vi "Delete Tags.vi"(8 "error in (no error)":errorcluster, 10 "Tag":string[](array[string]), 11 "Tag Tree In":refnum<class "Tag Tree.lvclass">) -> (0 "error out":errorcluster, 3 "Tag Tree Out":refnum<class "Tag Tree.lvclass">)   [LabVIEW 2020, in "Tag Tree.lvclass"]
uses:
  Tag Tree.lvclass
  Tag Tree.lvclass/Tag Tree.ctl
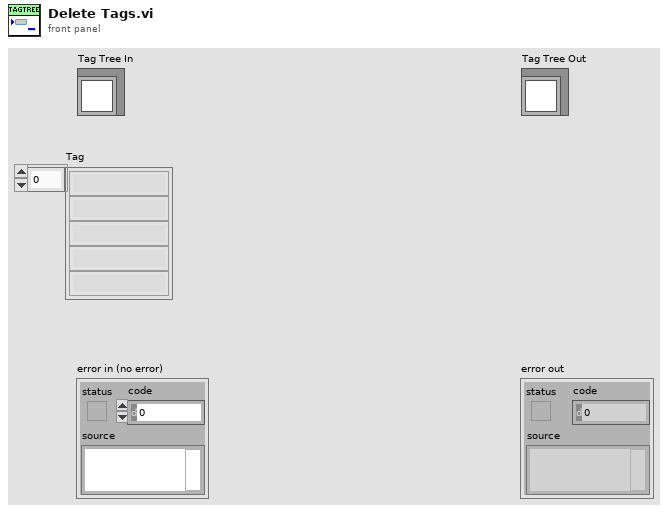
[diagram p1: front panel]
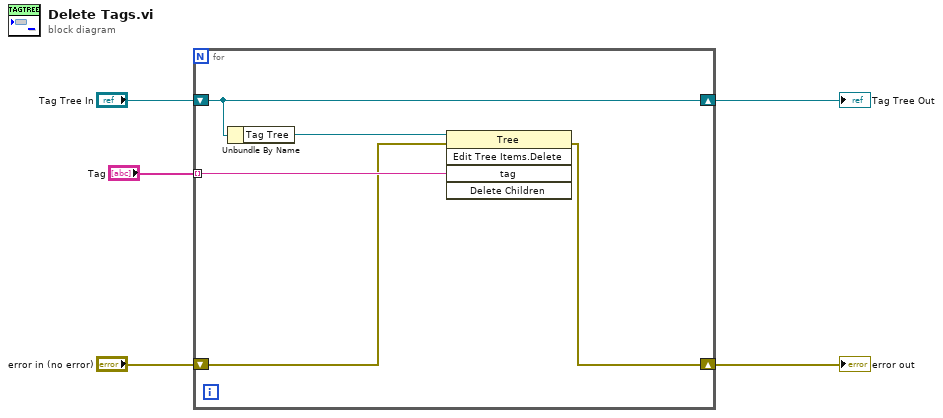
[diagram p0: block diagram]
diagram:
  n1 = for {
    tunnel: "Tag" -> [w9] mode=indexing
    shift-right: [w7] -> w2
    shift-left: "error in (no error)" -> [w8]
    shift-right: [w6] -> w1
    shift-left: "Tag Tree In" -> [w6]
    n2 = Unbundle By Name(w6) -> ("Tag Tree"=w10:refnum<vi>)
    n3 = invoke class="Tree" method="Edit Tree Items.Delete"(reference=w10, error in=w8, "tag"=w9) -> (error out=w7:errorcluster)  [unwired: 2 in, 4 out]
  }
  "error out" <- w2
  "Tag Tree Out" <- w1
